vi "Read MultCol Listbox Data.vi"(8 "error in":errorcluster, 11 "Multicolumn Listbox Ref in":refnum<vi>) -> (0 "error out":errorcluster, 1 "Interpret As Unicode":bool, 2 "Value":string[][](array[string]), 3 "Multicolumn Listbox Ref out":refnum<vi>)   [LabVIEW 2020, in "G-Unicode.lvlib"]
uses:
  Unicode/SubVIs/Byte Order Marks.vi
  G-Unicode.lvlib
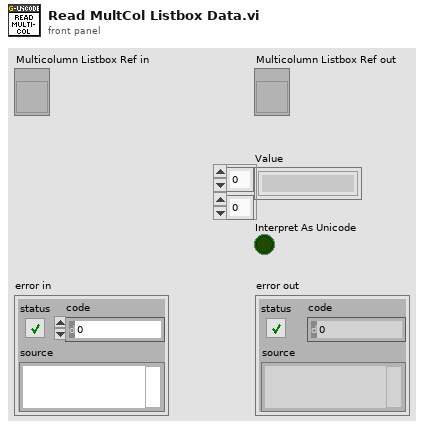
[diagram p1: front panel]
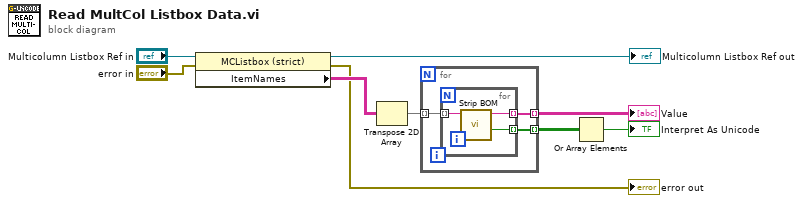
[diagram p0: block diagram]
diagram:
  n1 = property class="MCListbox (strict)"(reference="Multicolumn Listbox Ref in", error in="error in") -> (reference out=→"Multicolumn Listbox Ref out":refnum<vi>, error out=→"error out":errorcluster, "ItemNames"=w9:string[][])
  n2 = Transpose 2D Array(2D array=w9) -> (transposed array=w8:string[][])
  n3 = for {
    tunnel: w8 -> [w12] mode=indexing
    tunnel: [w11] -> w5 mode=indexing
    tunnel: [w10] -> w7 mode=indexing
    n4 = for {
      tunnel: w12 -> [w15] mode=indexing
      tunnel: [w14] -> w11 mode=indexing
      tunnel: [w13] -> w10 mode=indexing
      n5 = call "Strip BOM.vi"("String"=w15) -> ("BOM Found"=w13:bool, "String without BOM"=w14:string)  [unwired: 8 in, 1 out]
    }
  }
  "Value" <- w5
  n6 = Or Array Elements(Boolean array=w7) -> (logical OR=→"Interpret As Unicode":bool)
